vi "Init.vi"(8 "error in (no error)":errorcluster, 9 "Measurement Times":string[](array[string]), 10 "SA Pin":string, 11 "Measurement Name":string) -> (0 "error out":errorcluster, 3 "ModeSwitch Eval out":refnum<class "ModeSwitch Eval.lvclass">)   [LabVIEW 2016, in "SeqAuto Evaluations.lvlib" / "ModeSwitch Eval.lvclass"]
uses:
  ModeSwitch Eval.lvclass
  C:/Sequence Automation/Plugins/SeqAuto IEvaluation.lvlibp/SeqAuto IEvaluation.lvclass
  ModeSwitch Eval.lvclass/ModeSwitch Eval.ctl
  Plugins/SeqAuto IEvaluation.lvlibp/Write Measurement Name.vi
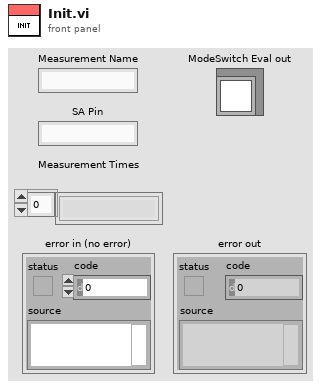
[diagram p1: front panel]
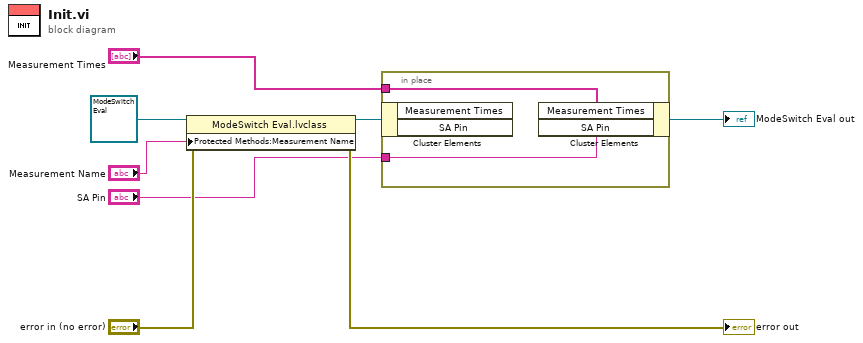
[diagram p0: block diagram]
diagram:
  n1 = property class="ModeSwitch Eval.lvclass"(reference=refnum<class "ModeSwitch Eval.lvclass"> refnum ("ModeSwitch Eval in"), error in="error in (no error)", "Protected Methods:Measurement Name"="Measurement Name") -> (reference out=w4:refnum<class "ModeSwitch Eval.lvclass">, error out=→"error out":errorcluster)
  n2 = in-place {
    in-place-border: "Measurement Times" -> [w10]
    in-place-border: "SA Pin" -> [w9]
    n3 = in-place-cluster #1(w4) -> ()  [unwired: 2 out]
    n4 = in-place-cluster #1("Measurement Times"=w10, "SA Pin"=w9) -> (→"ModeSwitch Eval out":refnum<class "ModeSwitch Eval.lvclass">)
  }
